vi "GetVision.vi"(5 "Turret_H (deg)":dbl, 7 "Pitch (deg)":dbl, 9 "Roll (deg)":dbl) -> (4 "LimeLight Raw Z Power Port (in)":dbl, 6 "LimeLight Raw X Power Port (in)":dbl, 8 "LimeLight Distance to Power Port (in)":dbl, 10 "LimeLight Raw Horizontal Offset Power Port (deg)":dbl, 12 "LimeLight Horizontal Offset to Ball (in)":dbl, 13 "LimeLight Raw Horizontal Offset to Ball (deg)":dbl, 14 "LimeLight Distance to Ball (in)":dbl, 15 "LimeLight Heading to Power Port (deg)":dbl)   [LabVIEW 2019]
doc: "This VI reads the raw data from the LimeLight pipeline and runs several validity checks. This VI calculates the current range and heading to either the Power Port or a Power Cell depending on the selected LimeLight pipeline."
uses:
  <vilib>/Rock Robotics/Network Tables/NT Read Number.vi
  <vilib>/Rock Robotics/Network Tables/NT Read Numeric Array.vi
  outputs.vi
  sensors.vi
  constants.vi
panel:
  in  "Maximum Pointing Error (deg)":dbl=15.0
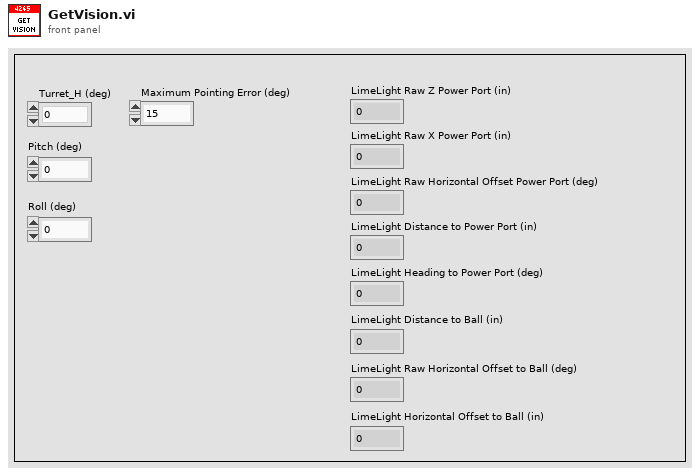
[diagram p1: front panel]
types:
  T1 = enum16{"Boot Up", "Camera Override", "Power Port", "Ball Tracking", "Transitioning"}
  T2 = enum16{"Boot Up", "Camera Override", "Power Port", "Ball Tracking"}
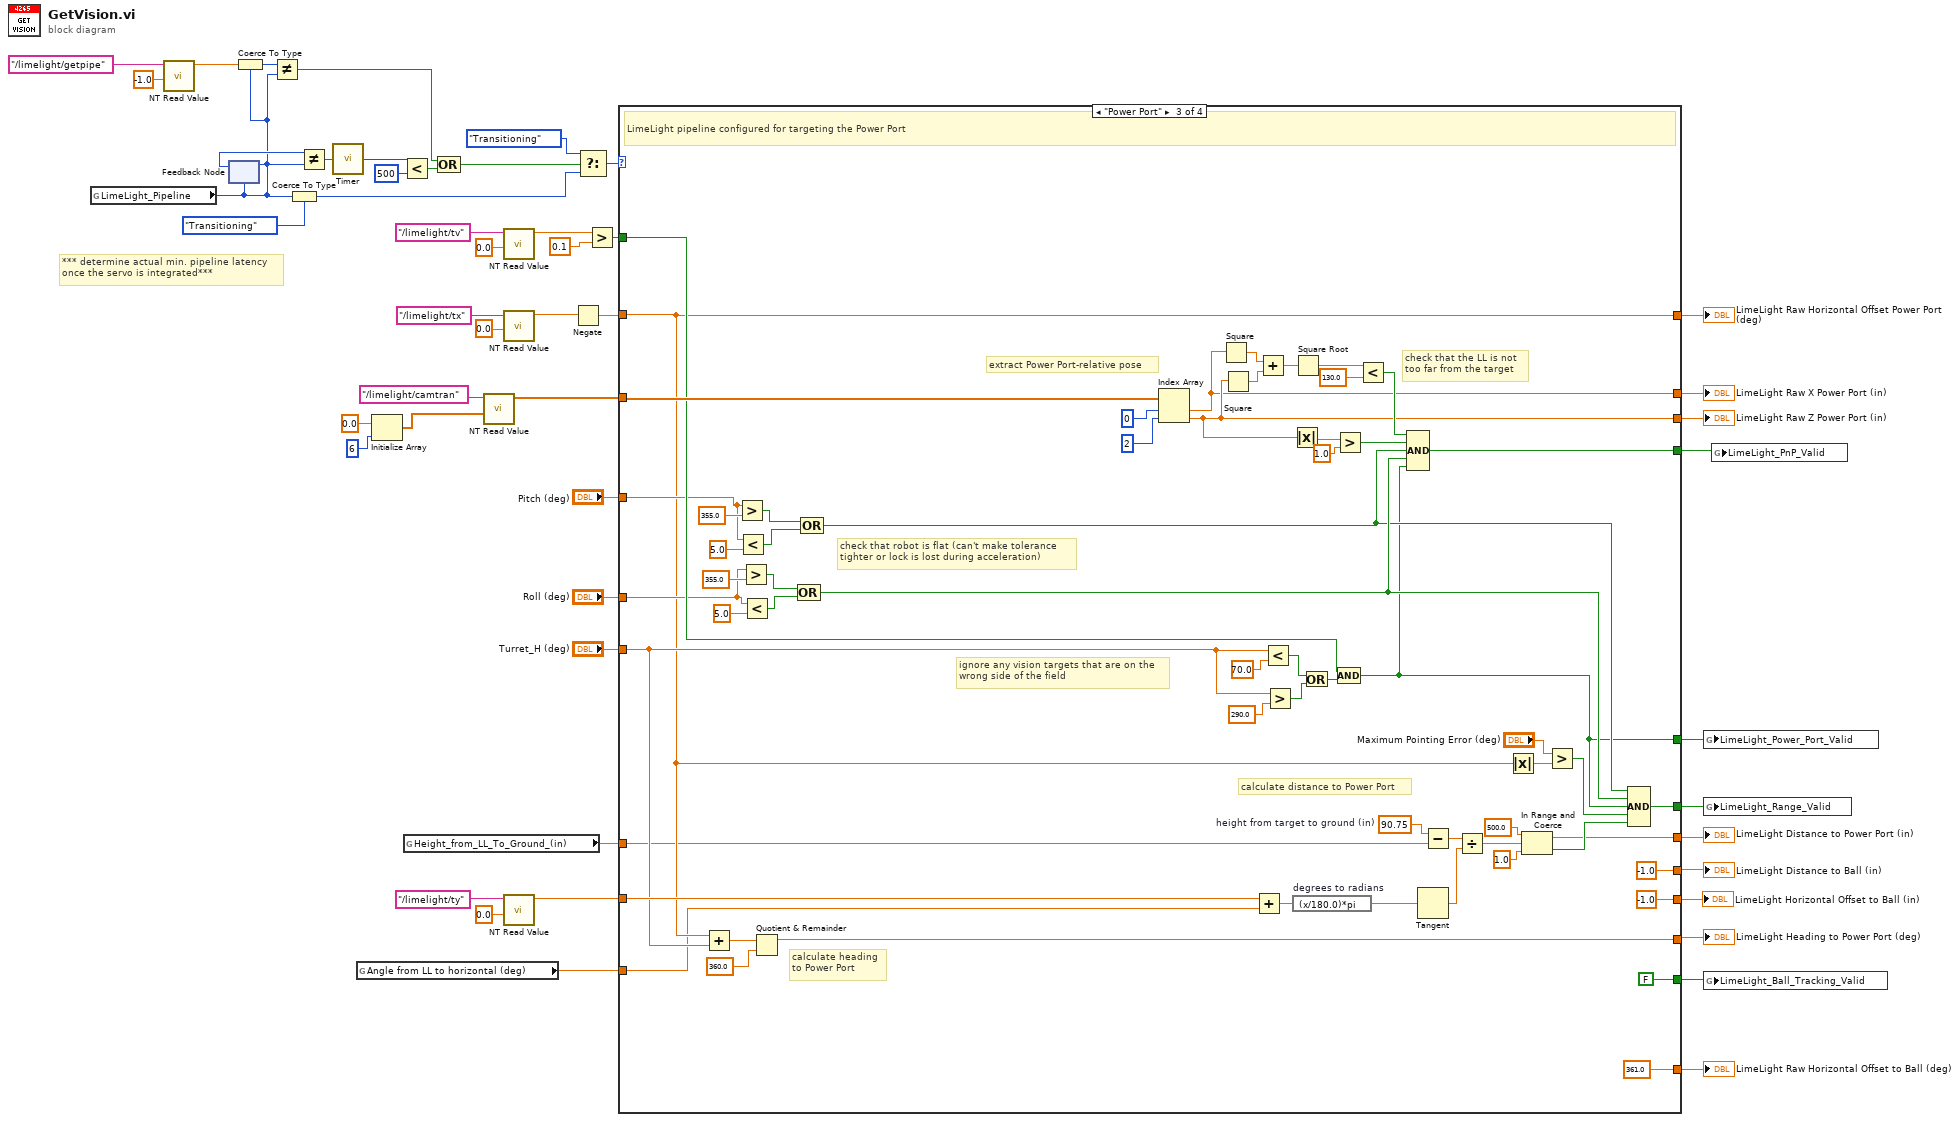
[diagram p0: block diagram]
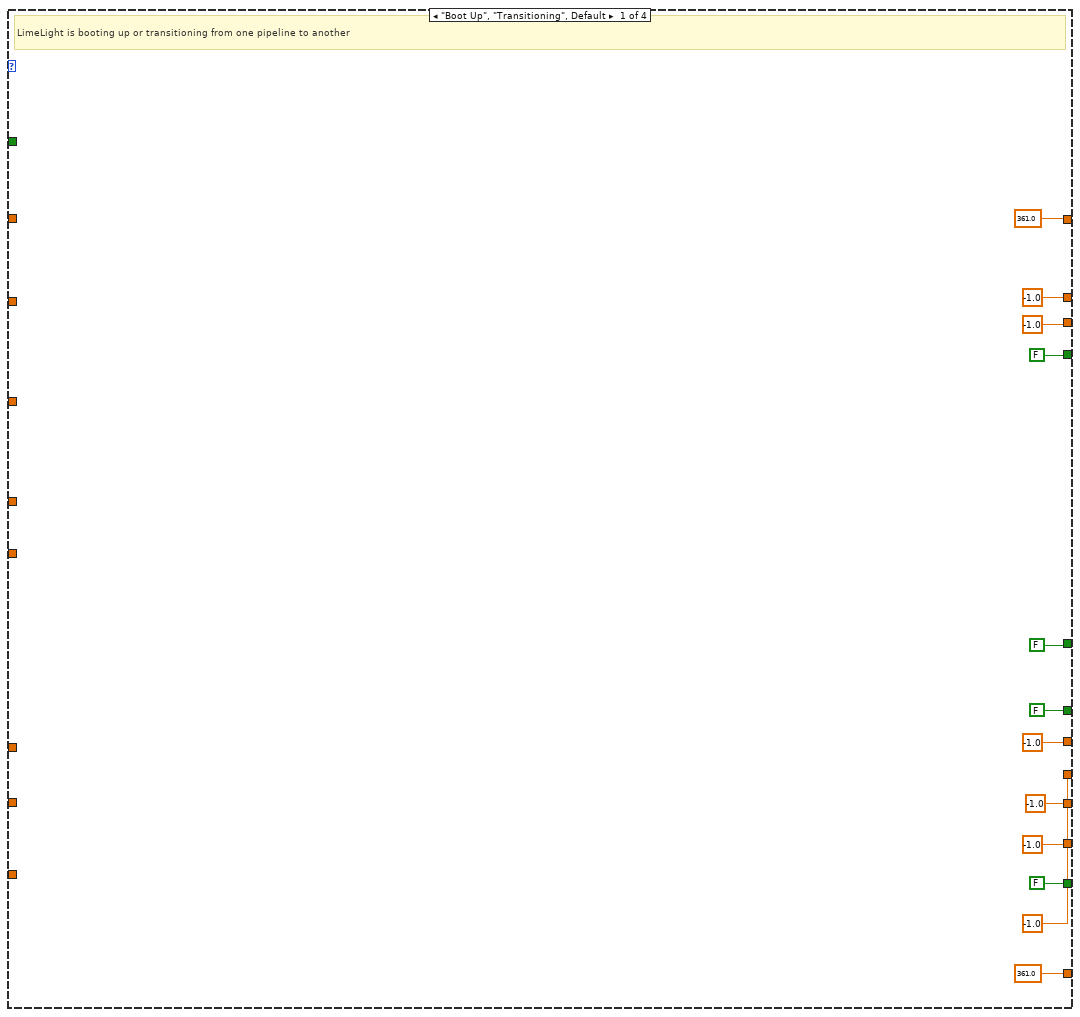
[diagram p2: hidden frame]
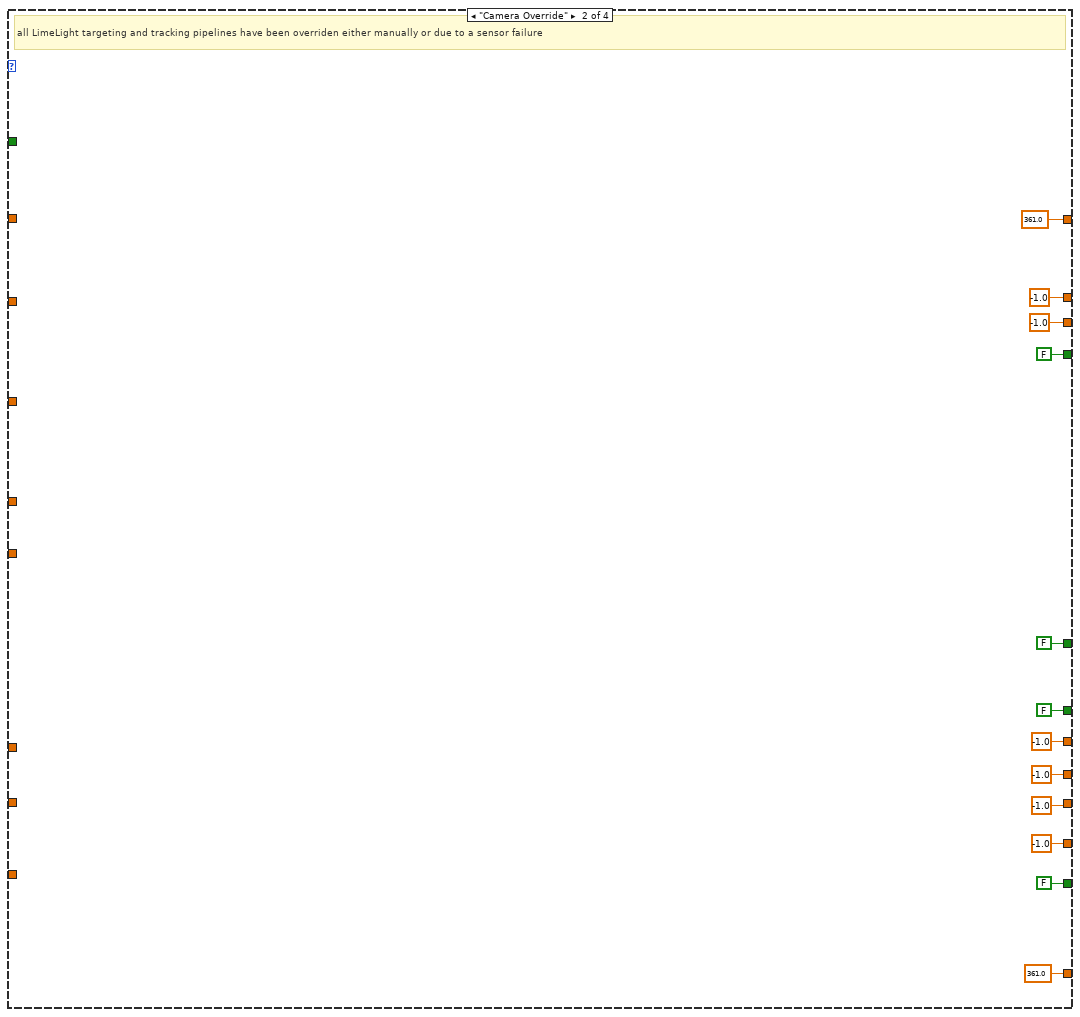
[diagram p3: hidden frame]
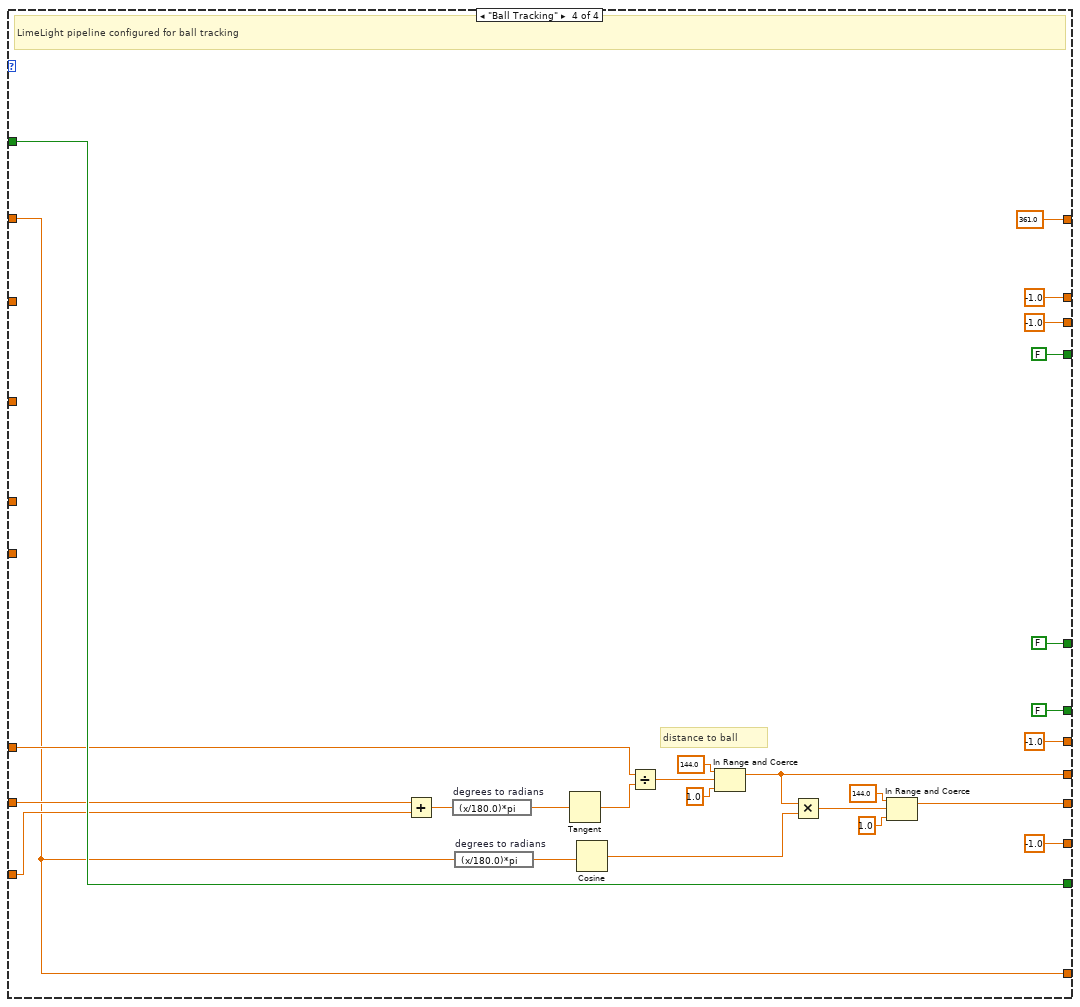
[diagram p4: hidden frame]
diagram:
  # "*** determine actual min. pipeline latency\nonce the servo is integrated***"
  n1 = global read "outputs.vi" "LimeLight_Pipeline"() -> (w6:T2)
  n2 = call-poly <vilib>:"NT Read Value.vi"("Default Value"=-1.0, "Name"="/limelight/getpipe") -> ("Numeric"=w7:dbl)  [unwired: 8 in, 1 out]
  n3 = feedback-in #1(w6) -> ()
  n4 = feedback #1(w6) -> (w21:T2)
  n5 = Coerce To Type(0:w7, 1:w6) -> (2:w8:T2)
  n6 = Not Equal?(x=w8, y=w6) -> (x != y?=w5:bool)
  n7 = Coerce To Type(0:w6, 1:T1."Transitioning") -> (2:w19:T1)
  n8 = Not Equal?(x=w21, y=w6) -> (x != y?=w25:bool)
  n9 = call "Timer.vi"("Reset Timer"=w25) -> ("Time (ms)"=w24:u32)
  n10 = global read "sensors.vi" "Angle from LL to horizontal (deg)"() -> (w3:dbl)
  n11 = Initialize Array(0.0 ("element"), 6 ("dimension size")) -> (w38:dbl[])
  n12 = Less?(x=w24, y=u32 500) -> (x < y?=w15:bool)
  n13 = global read "constants.vi" "Height_from_LL_To_Ground_(in)"() -> (w2:dbl)
  n14 = Compound Arithmetic op=OR(w5, w15) -> (w4:bool)
  n15 = call-poly <vilib>:"NT Read Value.vi"("Default Value"=w38, "Name"="/limelight/camtran") -> ("Numeric Array"=w34:dbl[])  [unwired: 8 in, 1 out]
  n16 = call-poly <vilib>:"NT Read Value.vi"("Default Value"=0.0, "Name"="/limelight/tv") -> ("Numeric"=w31:dbl)  [unwired: 8 in, 1 out]
  n17 = call-poly <vilib>:"NT Read Value.vi"("Default Value"=0.0, "Name"="/limelight/tx") -> ("Numeric"=w11:dbl)  [unwired: 8 in, 1 out]
  n18 = call-poly <vilib>:"NT Read Value.vi"("Default Value"=0.0, "Name"="/limelight/ty") -> ("Numeric"=w39:dbl)  [unwired: 8 in, 1 out]
  n19 = Negate(x=w11) -> (-x=w12:dbl)
  n20 = Select(t=T1."Transitioning", s=w4, f=w19) -> (s? t:f=w18:T1)
  n21 = Greater?(x=w31, y=0.1) -> (0:w27:bool)
  n22 = case shown="\"Power Port\"" w18 {
    tunnel: "Turret_H (deg)" -> [_ _ w81 _]
    tunnel: [FALSE FALSE w94 FALSE] -> w49
    tunnel: [FALSE FALSE w93 FALSE] -> w48
    tunnel: [FALSE FALSE w92 FALSE] -> w47
    tunnel: [-1.0 ("upper limit") -1.0 ("upper limit") w91 -1.0 ("upper limit")] -> w46
    tunnel: [-1.0 ("Numeric") -1.0 ("Numeric") w90 -1.0 ("Numeric")] -> w45
    tunnel: [-1.0 ("Numeric") -1.0 ("Numeric") w89 -1.0 ("Numeric")] -> w44
    tunnel: [-1.0 -1.0 w88 -1.0] -> w43
    tunnel: [361.0 361.0 w78 361.0] -> w42
    tunnel: w39 -> [_ _ w87 w148]
    tunnel: w34 -> [_ _ w86 _]
    tunnel: w12 -> [_ _ w78 w139]
    tunnel: w27 -> [_ _ w82 w152]
    tunnel: [FALSE FALSE FALSE w152] -> w26
    tunnel: [-1.0 ("upper limit") -1.0 ("upper limit") -1.0 ("upper limit") w142] -> w17
    tunnel: [361.0 361.0 361.0 w139] -> w16
    tunnel: "Roll (deg)" -> [_ _ w80 _]
    tunnel: "Pitch (deg)" -> [_ _ w79 _]
    tunnel: w3 -> [_ _ w77 w147]
    tunnel: w2 -> [_ _ w76 w143]
    tunnel: [-1.0 ("upper limit") -1.0 ("upper limit") -1.0 ("upper limit") w135] -> w1
    frame "Boot Up", "Transitioning", Default {
      # "LimeLight is booting up or transitioning from one pipeline to another"
    }
    frame "Camera Override" {
      # "all LimeLight targeting and tracking pipelines have been overriden either manually or due to a sensor failure"
    }
    frame "Power Port" {
      w118 = 90.75  # height from target to ground (in)
      # "check that robot is flat (can't make tolerance\ntighter or lock is lost during acceleration)"
      # "calculate heading\nto Power Port"
      # "calculate distance to Power Port"
      # "check that the LL is not\ntoo far from the target"
      # "extract Power Port-relative pose"
      # "ignore any vision targets that are on the\nwrong side of the field"
      # "LimeLight pipeline configured for targeting the Power Port"
      n23 = Add(x=w78, y=w81) -> (x+y=w113:dbl)
      n24 = Greater?(x=w79, y=355.0) -> (0:w103:bool)
      n25 = Less?(x=w79, y=5.0) -> (x < y?=w102:bool)
      n26 = Greater?(x=w80, y=355.0) -> (0:w99:bool)
      n27 = Less?(x=w80, y=5.0) -> (x < y?=w98:bool)
      n28 = Quotient & Remainder(x=w113, y=360.0) -> (x-y*floor(x/y)=w88:dbl)  [unwired: 1 out]
      n29 = Compound Arithmetic op=OR(w99, w98) -> (w96:bool)
      n30 = Compound Arithmetic op=OR(w103, w102) -> (w95:bool)
      n31 = Index Array(array=w86, index #1=0 ("index"), index #2=2 ("index")) -> (element #1=w89:dbl, element #2=w90:dbl)
      n32 = Square(x=w89) -> (x^2=w124:dbl)
      n33 = Square(x=w90) -> (x^2=w123:dbl)
      n34 = Add(x=w87, y=w77) -> (x+y=w116:dbl)
      n35 = Add(x=w124, y=w123) -> (x+y=w122:dbl)
      n36 = Less?(x=w81, y=70.0) -> (x < y?=w127:bool)
      n37 = Greater?(x=w81, y=290.0) -> (0:w128:bool)
      n38 = Absolute Value(x=w90) -> (abs(x)=w132:dbl)
      n39 = Square Root(x=w122) -> (sqrt(x)=w121:dbl)
      n40 = expression code="(x/180.0)*pi" "degrees to radians"(w116) -> (w115:dbl)
      n41 = Or(x=w127, y=w128) -> (x .or. y?=w125:bool)
      n42 = Greater?(x=w132, y=1.0) -> (0:w126:bool)
      n43 = Compound Arithmetic op=AND(w82, w125) -> (w93:bool)
      n44 = Less?(x=w121, y=130.0) -> (x < y?=w119:bool)
      n45 = Compound Arithmetic op=AND(w119, w126, w95, w96, w93) -> (w92:bool)
      n46 = Tangent(1:w115) -> (0:w114:dbl)
      n47 = Subtract(x=w118, y=w76) -> (x-y=w117:dbl)
      n48 = Divide(x=w117, y=w114) -> (x/y=w111:dbl)
      n49 = Absolute Value(x=w78) -> (abs(x)=w107:dbl)
      n50 = In Range and Coerce(upper limit=500.0, x=w111, lower limit=1.0) -> (coerced(x)=w91:dbl, In Range?=w108:bool)
      n51 = Greater?(x="Maximum Pointing Error (deg)", y=w107) -> (0:w97:bool)
      n52 = Compound Arithmetic op=AND(w95, w96, w93, w97, w108) -> (w94:bool)
    }
    frame "Ball Tracking" {
      # "distance to ball"
      # "LimeLight pipeline configured for ball tracking"
      n53 = Add(x=w148, y=w147) -> (x+y=w151:dbl)
      n54 = expression code="(x/180.0)*pi" "degrees to radians"(w151) -> (w150:dbl)
      n55 = expression code="(x/180.0)*pi" "degrees to radians"(w139) -> (w140:dbl)
      n56 = Tangent(1:w150) -> (0:w149:dbl)
      n57 = Cosine(x=w140) -> (cos(x)=w141:dbl)
      n58 = Divide(x=w143, y=w149) -> (x/y=w144:dbl)
      n59 = In Range and Coerce(upper limit=144.0, x=w144, lower limit=1.0) -> (coerced(x)=w142:dbl)  [unwired: 1 out]
      n60 = Multiply(x=w142, y=w141) -> (x*y=w137:dbl)
      n61 = In Range and Coerce(upper limit=144.0, x=w137, lower limit=1.0) -> (coerced(x)=w135:dbl)  [unwired: 1 out]
    }
  }
  "LimeLight Distance to Power Port (in)" <- w46
  "LimeLight Raw X Power Port (in)" <- w44
  "LimeLight Raw Z Power Port (in)" <- w45
  "LimeLight Heading to Power Port (deg)" <- w43
  "LimeLight Raw Horizontal Offset Power Port (deg)" <- w42
  "LimeLight Distance to Ball (in)" <- w17
  "LimeLight Raw Horizontal Offset to Ball (deg)" <- w16
  "LimeLight Horizontal Offset to Ball (in)" <- w1
  n62 = global write "sensors.vi" "LimeLight_Power_Port_Valid"(w48) -> ()
  n63 = global write "sensors.vi" "LimeLight_Range_Valid"(w49) -> ()
  n64 = global write "sensors.vi" "LimeLight_Ball_Tracking_Valid"(w26) -> ()
  n65 = global write "sensors.vi" "LimeLight_PnP_Valid"(w47) -> ()
